vi "Configuration Tool Main.vi"() -> ()   [LabVIEW 2014, in "Advanced Configuration Tool.lvlib"]
doc: "This is the main VI for the configuration editor."
uses:
  Advanced Configuration Tool.lvlib
  Controls/StateCluster.ctl
  <vilib>/NI/Configuration Framework/Repository/NISE_CEF_Repository.lvclass
  <vilib>/NI/Configuration Framework/Node/NodeRef.ctl
  <vilib>/NI/Configuration Framework/Node/NISE_CEF_Node.lvclass
  <vilib>/NI/Configuration Framework/Node/UserEventRef.ctl
  <vilib>/NI/Configuration Framework/Controls/EventCluster.ctl
  Controls/AddMessage.ctl
  Controls/MoveMessage.ctl
  <vilib>/Utility/error.llb/DialogType.ctl
  <vilib>/NI/Configuration Framework/hierarchy repo/NISE_CEF_HierarchyRepo.lvclass
  Classes/My System/My System.lvclass
  <vilib>/NI/AMC/Read Termination Message.vi
  <vilib>/NI/AMC/Create Single Message.vi
  <vilib>/NI/AMC/Update Message Routing Info.vi
  <vilib>/NI/AMC/Globals.vi
  <vilib>/NI/AMC/Send Message.vi
  <vilib>/NI/AMC/AMC.lvlib
  <vilib>/NI/Configuration Framework/NISE_CEF_TreeControl.lvlib
  <vilib>/NI/Configuration Framework/serializable configuration/NISE_CEF_serializable configuration.lvclass
panel:
  in  "View":string(tree)
  in  "Exit":bool
  # "Configurator"
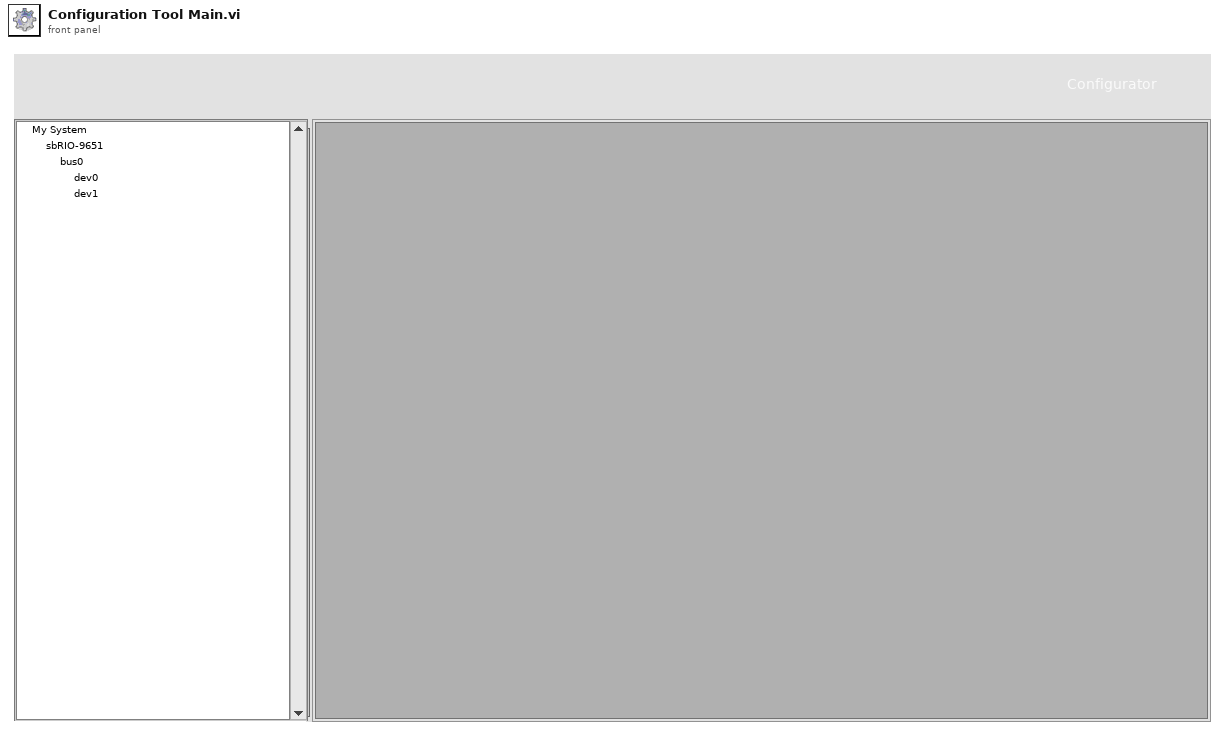
[diagram p1: front panel]
types:
  T1 = typedef "Advanced Configuration Tool.lvlib/StateCluster.ctl" = cluster{"repository":refnum<class "NISE_CEF_Repository.lvclass">, "root":T2, "unsaved changes":bool, "current path":path, "user event ref":T3, "glyph path":path, "classes path":path}
  T2 = typedef "NISE_CEF_Node.lvclass/NodeRef.ctl" = refnum<data-value>
  T3 = typedef "NISE_CEF_Node.lvclass/UserEventRef.ctl" = refnum<user-event>
  T4 = typedef "AMC.lvlib/Message Queue.ctl" = refnum<queue>
  T5 = typedef "Advanced Configuration Tool.lvlib/AddMessage.ctl" = cluster{"node type":string, "to add to":string}
  T6 = typedef "Advanced Configuration Tool.lvlib/MoveMessage.ctl" = cluster{"node ref":T2, "new parent":T2}
  T7 = enum32{"Invalid", "Standard", "Closed", "Hidden", "Minimized", "Maximized"}
  T8 = typedef "NISE_CEF_TreeControl.lvlib/EventCluster.ctl" = cluster{"command":string, "data":string}
  T9 = typedef "Advanced Configuration Tool.lvlib/FilePaths.ctl" = cluster{"glyphs":path, "classes":path}
  T10 = typedef "DialogType.ctl" = u16
  T11 = typedef "NISE_CEF_Node.lvclass/Summary.ctl" = cluster{"ID":string, "parent ID":string, "node type":string, "text":string, "additional text":string, "glyph":string, "depth":i32}
  T12 = typedef "LVPoint32TypeDef.ctl" = cluster{"Horizontal":i32, "Vertical":i32}
  T13 = cluster{"data name":string, "drag data":variant}[]
  T14 = typedef "NISE_CEF_Node.lvclass/NodeMenuOptions.ctl" = cluster{"removable":bool, "movable":bool, "duplicate":bool}
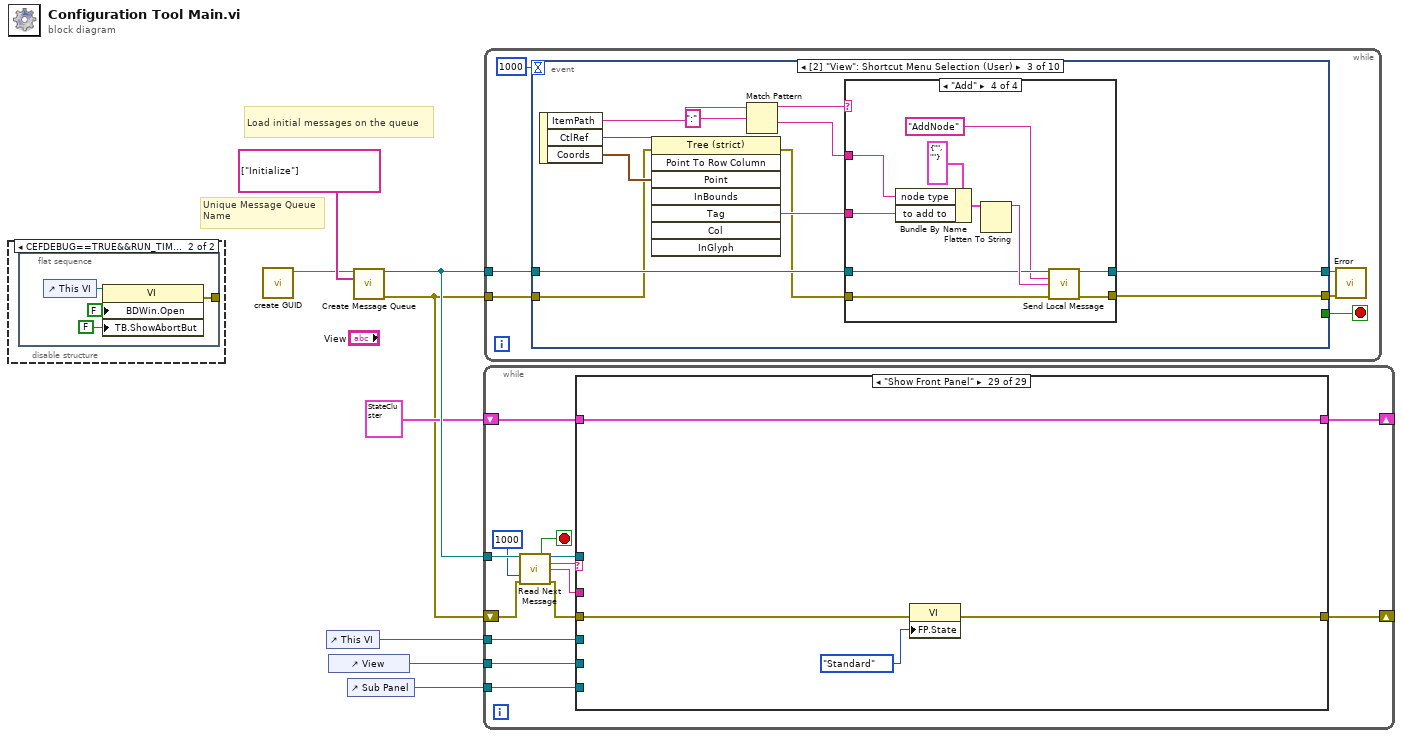
[diagram p0: block diagram]
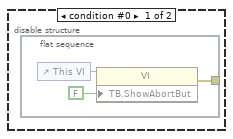
[diagram p2: hidden frame]
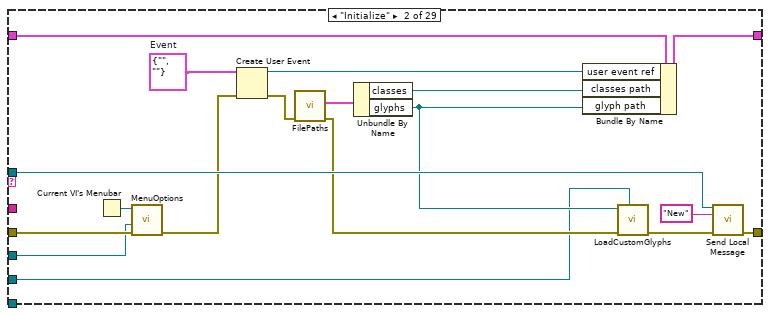
[diagram p4: hidden frame]
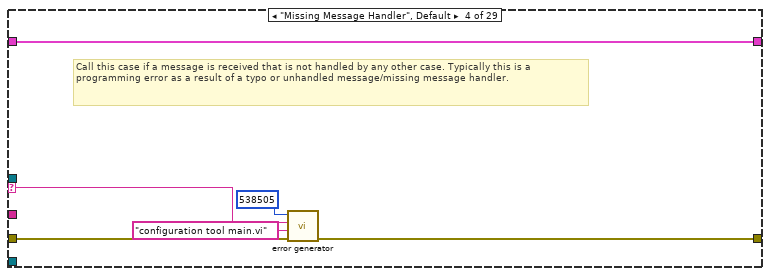
[diagram p6: hidden frame]
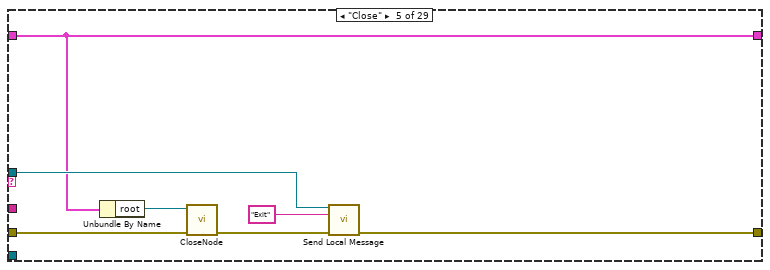
[diagram p7: hidden frame]
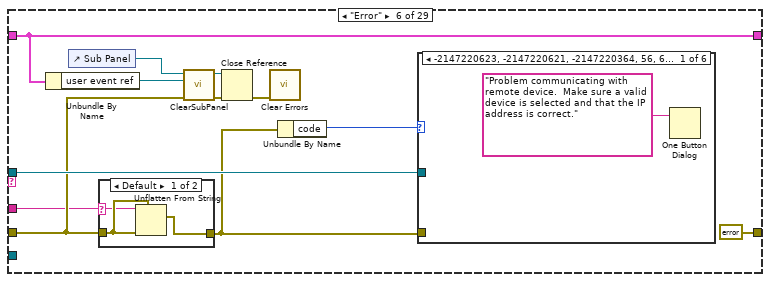
[diagram p8: hidden frame]
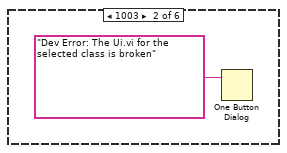
[diagram p10: hidden frame]
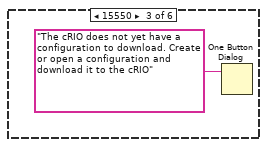
[diagram p11: hidden frame]
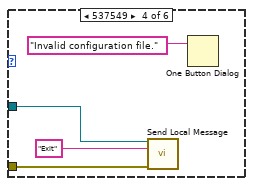
[diagram p12: hidden frame]
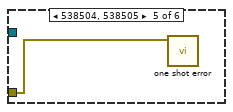
[diagram p13: hidden frame]
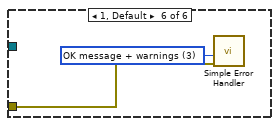
[diagram p14: hidden frame]
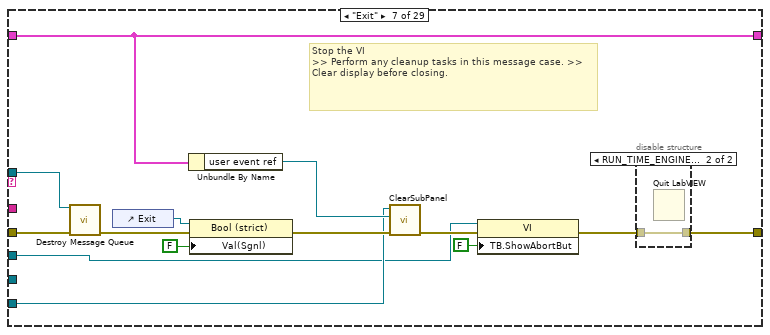
[diagram p15: hidden frame]
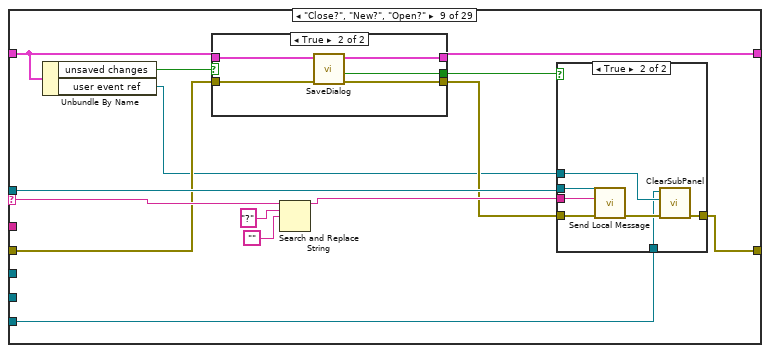
[diagram p18: hidden frame]
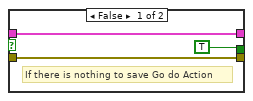
[diagram p19: hidden frame]
diagram:
  # "Unique Message Queue Name"
  # "Load initial messages on the queue"
  n1 = disable-structure shown="CEFDEBUG==TRUE&&RUN_TIME_ENGINE==False" {
    frame condition #0 {
      n2 = flat-sequence {
        tunnel: [w9] -> _
        frame #0 {
          n3 = control-ref of="This VI"() -> (w10:refnum<vi>)
          n4 = property class="VI"(reference=w10, "TB.ShowAbortBut"=FALSE ("Tool Bar:Show Abort Button")) -> (error out=w9:errorcluster)  [unwired: 1 in, 1 out]
        }
      }
    }
    frame condition #1 (active) {
      n5 = flat-sequence {
        tunnel: [w14] -> _
        frame #0 {
          n6 = control-ref of="This VI"() -> (w15:refnum<vi>)
          n7 = property class="VI"(reference=w15, "BDWin.Open"=FALSE ("Block Diagram Window:Open"), "TB.ShowAbortBut"=FALSE ("Tool Bar:Show Abort Button")) -> (error out=w14:errorcluster)  [unwired: 1 in, 1 out]
        }
      }
    }
  }
  n8 = call <vilib>:"create GUID.vi"() -> ("uuid"=w2:string)  [unwired: 11 in]
  n9 = control-ref of="This VI"() -> (w4:refnum<vi>)
  n10 = control-ref of="View"() -> (w3:refnum<vi>)
  n11 = control-ref of="Sub Panel"() -> (w1:refnum<vi>)
  n12 = call <vilib>:"Create Message Queue.vi"("message queue name"=w2, "initial message names"=string[] ["Initialize"]) -> ("message queue out"=w7:T4, "error out"=w5:errorcluster)  [unwired: 12 in]
  n13 = while "Message Processor" {
    shift-right: [w25] -> _
    shift-left: w5 -> [w24]
    tunnel: w7 -> [w23]
    shift-right: [w21] -> _
    shift-left: T1 {"repository"=refnum, "root"=refnum, "unsaved changes"=FALSE, "current path"=path "", "user event ref"=refnum, "glyph path"=path "", "classes path"=path ""} -> [w20]
    tunnel: w4 -> [w18]
    tunnel: w3 -> [w17]
    tunnel: w1 -> [w16]
    stop <- w29 stop-if-true
    n14 = call <vilib>:"Read Next Message.vi"("message queue in"=w23, "timeout (1 ms)"=1000, "error in"=w24) -> ("exit process?"=w29:bool, "message queue out"=w19:T4, "message name"=w28:string, "message value"=w27:string, "error out"=w26:errorcluster)  [unwired: 5 in, 3 out]
    n15 = case shown="\"Show Front Panel\"" w28 {
      selector: w28 -> [_ _ _ w54 _ _ _ _ w118 _ _ _ _ _ _ _ _ _ _ w366 _ _ _ _ _ _ _ _ _]
      tunnel: w27 -> [_ _ _ _ _ w65 _ _ _ _ _ _ _ w240 w272 _ w300 w332 w346 w364 w404 w428 _ _ w471 w493 _ _ _]
      tunnel: w26 -> [w31 w49 w51 w56 w59 w68 w104 w108 w111 w155 w166 w206 w232 w247 w273 w290 w301 w322 w345 w369 w406 w427 w452 w461 w470 w491 w496 w498 w503]
      tunnel: [w31 w45 w51 w55 w63 errorcluster {"status"=FALSE, "code"=0, "source"=""} ("error out") w97 w108 w122 w146 w162 w210 w234 w244 w260 w290 w304 w324 w349 w372 w410 w424 w447 w456 w467 w486 w496 w497 w502] -> w25
      tunnel: [w30 w40 w50 w57 w61 w73 w96 w107 w113 w159 w167 w213 w233 w241 w269 w289 w307 w315 w342 w373 w408 w421 w454 w460 w465 w482 w495 w500 w504] -> w21
      tunnel: w20 -> [w30 w41 w50 w57 w61 w73 w96 w107 w114 w158 w168 w208 w231 w242 w270 w289 w303 w320 w350 w373 w409 w429 w454 w460 w465 w494 w495 w500 w504]
      tunnel: w19 -> [_ w44 _ _ w62 w76 w103 _ w121 w160 w164 w209 _ w243 w265 _ w291 _ _ w367 _ _ _ _ w466 w485 _ _ _]
      tunnel: w18 -> [_ w32 _ _ _ _ w92 _ _ _ _ _ _ _ _ _ _ _ _ _ _ _ w439 _ _ _ _ _ _]
      tunnel: w17 -> [_ w33 _ _ _ _ _ _ _ _ _ _ _ _ _ _ _ w316 w343 w361 w401 w422 w440 _ _ _ _ _ _]
      tunnel: w16 -> [_ _ _ _ _ _ w94 _ w109 _ _ _ _ _ _ _ _ _ _ _ _ _ w437 w455 w462 _ _ _ _]
      frame "------------Generic Operations------------" {
        # "Dummy case to add a seperation in the Case Structure menu"
      }
      frame "Initialize" {
        w35 = T8 {"command"="", "data"=""}  # Event
        n16 = Current VI's Menubar() -> (w48:refnum<k9>)
        n17 = call "MenuOptions.vi"("error in"=w49, "VI ref"=w32, "menu ref in"=w48) -> ("error out"=w39:errorcluster)  [unwired: 7 in, 1 out]
        n18 = Create User Event(user event datatype=w35, error in=w39) -> (user event=w34:refnum<user-event>, error out=w38:errorcluster)
        n19 = call "FilePaths.vi"("error in"=w38) -> ("error out"=w43:errorcluster, "paths"=w42:T9)  [unwired: 9 in]
        n20 = Unbundle By Name(w42) -> ("classes"=w37:path, "glyphs"=w36:path)
        n21 = Bundle By Name(cluster=w41, "user event ref"=w34, "classes path"=w37, "glyph path"=w36) -> (w40:T1)
        n22 = call <vilib>:"LoadCustomGlyphs.vi"("tree ref"=w33, "error in"=w43, "glyph directory"=w36) -> ("error out"=w46:errorcluster)  [unwired: 8 in]
        n23 = call <vilib>:"Send Local Message.vi"("message queue in"=w44, "message name"="New" ("Message Name"), "error in"=w46) -> ("error out"=w45:errorcluster)  [unwired: 10 in, 2 out]
      }
      frame "", "Idle" {
      }
      frame "Missing Message Handler", Default {
        # "Call this case if a message is received that is not handled by any other case. Typically this is a programming error as a result of a typo or unhandled message/missing message handler."
        n24 = call <vilib>:"error generator.vi"("error in"=w56, "source"="configuration tool main.vi", "append error message"=w54, "error code (0)"=538505) -> ("error out"=w55:errorcluster)  [unwired: 5 in]
      }
      frame "Close" {
        n25 = Unbundle By Name(w61) -> ("root"=w60:T2)
        n26 = call <vilib>:"CloseNode.vi"("error in"=w59, "node ref"=w60) -> ("error out"=w58:errorcluster)  [unwired: 9 in]
        n27 = call <vilib>:"Send Local Message.vi"("message queue in"=w62, "message name"="Exit", "error in"=w58) -> ("error out"=w63:errorcluster)  [unwired: 10 in, 2 out]
      }
      frame "Error" {
        n28 = Unbundle By Name(w73) -> ("user event ref"=w71:T3)
        n29 = control-ref of="Sub Panel"() -> (w72:refnum<vi>)
        n30 = case shown="Default" w65 {
          selector: w65 -> [w78 _]
          tunnel: w68 -> [w79 w80]
          tunnel: [w77 w80] -> w67
          frame Default {
            n31 = Unflatten From String(type=w79, binary string=w78, error in (no error)=w79) -> (value=w77:errorcluster)  [unwired: 2 in, 2 out]
          }
          frame "" {
          }
        }
        n32 = call <vilib>:"ClearSubPanel.vi"("error in"=w68, "user event ref"=w71, "sub panel ref in"=w72) -> ("error out"=w70:errorcluster, "sub panel ref out"=w69:refnum<vi>)  [unwired: 7 in]
        n33 = Close Reference(reference=w69, error in (no error)=w70) -> (error out=w66:errorcluster)
        n34 = call <vilib>:"Clear Errors.vi"("error in (no error)"=w66) -> ()  [unwired: 5 in, 2 out]
        n35 = Unbundle By Name(w67) -> ("code"=w74:i32)
        n36 = case shown="-2147220623, -2147220621, -2147220364, 56, 63" w74 {
          tunnel: w76 -> [_ _ _ w86 _ _]
          tunnel: w67 -> [_ _ _ w85 w88 w90]
          frame -2147220623, -2147220621, -2147220364, 56, 63 {
            n37 = One Button Dialog(message="Problem communicating with remote device.  Make sure a valid device is selected and that the IP address is correct.") -> ()  [unwired: 1 in, 1 out]
          }
          frame 1003 {
            n38 = One Button Dialog(message="Dev Error: The Ui.vi for the selected class is broken") -> ()  [unwired: 1 in, 1 out]
          }
          frame 15550 {
            n39 = One Button Dialog(message="The cRIO does not yet have a configuration to download. Create or open a configuration and download it to the cRIO") -> ()  [unwired: 1 in, 1 out]
          }
          frame 537549 {
            n40 = call <vilib>:"Send Local Message.vi"("message queue in"=w86, "message name"="Exit", "error in"=w85) -> ()  [unwired: 10 in, 3 out]
            n41 = One Button Dialog(message="Invalid configuration file.") -> ()  [unwired: 1 in, 1 out]
          }
          frame 538504, 538505 {
            n42 = call <vilib>:"one shot error.vi"("error in"=w88) -> ()  [unwired: 11 in]
          }
          frame 1, Default {
            w89 = T10 3 items=["no dialog", "OK message", "continue or stop message", "OK message + warnings", "continue/stop + warnings"] ("type of dialog (OK msg:1)")
            n43 = call <vilib>:"Simple Error Handler.vi"("type of dialog (OK msg:1)"=w89, "error in (no error)"=w90) -> ()  [unwired: 8 out]
          }
        }
      }
      frame "Exit" {
        # "Stop the VI                                                                             >> Perform any cleanup tasks in this message case. >> Clear display before closing."
        n44 = call <vilib>:"Destroy Message Queue.vi"("message queue in"=w103, "error in"=w104) -> ("error out"=w100:errorcluster)  [unwired: 11 in, 2 out]
        n45 = control-ref of="Exit"() -> (w102:refnum<vi>)
        n46 = Unbundle By Name(w96) -> ("user event ref"=w95:T3)
        n47 = property class="Bool (strict)"(reference=w102, error in=w100, "Val(Sgnl)"=FALSE ("Exit")) -> (error out=w99:errorcluster)  [unwired: 1 out]
        n48 = call <vilib>:"ClearSubPanel.vi"("error in"=w99, "user event ref"=w95, "sub panel ref in"=w94) -> ("error out"=w98:errorcluster)  [unwired: 7 in, 1 out]
        n49 = property class="VI"(reference=w92, error in=w98, "TB.ShowAbortBut"=FALSE ("Tool Bar:Show Abort Button")) -> (error out=w93:errorcluster)  [unwired: 1 out]
        n50 = disable-structure shown="RUN_TIME_ENGINE==True" {
          disable-tunnel: [w105 w106] -> w97
          disable-tunnel: w93 -> [w105 w106]
          frame condition #0 (active) {
          }
          frame condition #1 {
            n51 = Quit LabVIEW() -> ()  [unwired: 1 in]
          }
        }
      }
      frame "------------Menu Operations--------------" {
        # "Dummy case to add a seperation in the Case Structure menu"
      }
      frame "Close?", "New?", "Open?" {
        n52 = Unbundle By Name(w114) -> ("unsaved changes"=w116:bool, "user event ref"=w110:T3)
        n53 = case shown="True" w116 {
          tunnel: [TRUE ("SaveFlag") w130] -> w115
          tunnel: w114 -> [w124 w129]
          tunnel: [w124 w128] -> w113
          tunnel: w111 -> [w123 w127]
          tunnel: [w123 w126] -> w112
          frame False {
            # "If there is nothing to save Go do Action"
          }
          frame True {
            n54 = call "SaveDialog.vi"("error in"=w127, "state in"=w129) -> ("error out"=w126:errorcluster, "new"=w130:bool, "state out"=w128:T1)  [unwired: 7 in]
          }
        }
        n55 = Search and Replace String(input string=w118, search string="?", replace string="") -> (result string=w117:string)  [unwired: 5 in, 3 out]
        n56 = case shown="True" w115 {
          tunnel: w112 -> [w131 w138]
          tunnel: [w131 w134] -> w122
          tunnel: w121 -> [_ w137]
          tunnel: w117 -> [_ w136]
          tunnel: w110 -> [_ w133]
          tunnel: w109 -> [_ w132]
          frame False {
          }
          frame True {
            n57 = call <vilib>:"Send Local Message.vi"("message queue in"=w137, "message name"=w136, "error in"=w138) -> ("error out"=w135:errorcluster)  [unwired: 10 in, 2 out]
            n58 = call <vilib>:"ClearSubPanel.vi"("error in"=w135, "user event ref"=w133, "sub panel ref in"=w132) -> ("error out"=w134:errorcluster)  [unwired: 7 in, 1 out]
          }
        }
      }
      frame "New" {
        n59 = Unbundle By Name(w158) -> ("classes path"=w157:path)
        n60 = call-dynamic "Initialize.vi"("error in"=w155, "path"=w157, "repository in"=refnum<class "NISE_CEF_HierarchyRepo.lvclass"> refnum ("NISE_CEF_HierarchyRepo.lvclass")) -> ("error out"=w156:errorcluster, "repository out"=w149:refnum<class "NISE_CEF_HierarchyRepo.lvclass">)  [unwired: 7 in]
        n61 = call-dynamic "Initialize.vi"("error in"=w156, "node in"=refnum<class "My System.lvclass"> refnum ("My System.lvclass")) -> ("error out"=w143:errorcluster, "data value reference"=w144:T2)  [unwired: 7 in, 1 out]
        n62 = call <vilib>:"NodetoID.vi"("error in"=w143, "node ref"=w144) -> ("error out"=w142:errorcluster, "ID"=w140:string)  [unwired: 8 in]
        n63 = call <vilib>:"Send Local Message.vi"("message queue in"=w160, "message name"="PopulateTree", "error in"=w142) -> ("message queue out"=w145:T4, "error out"=w151:errorcluster)  [unwired: 10 in, 1 out]
        n64 = Current VI's Menubar() -> (w150:refnum<k9>)
        n65 = call <vilib>:"NewMenu.vi"("error in"=w151, "menu ref in"=w150, "NISE_CEF_Repository in"=w149) -> ("error out"=w147:errorcluster, "NISE_CEF_Repository out"=w148:refnum<class "NISE_CEF_HierarchyRepo.lvclass">)  [unwired: 6 in, 1 out]
        n66 = Bundle By Name(cluster=w158, "current path"=path "", "unsaved changes"=FALSE, "repository"=w148, "root"=w144) -> (w159:T1)
        n67 = call <vilib>:"Send Local Message.vi"("message queue in"=w145, "message name"="ActivateNode", "message value"=w140, "error in"=w147) -> ("error out"=w146:errorcluster)  [unwired: 9 in, 2 out]
      }
      frame "Open" {
        n68 = in-place {
          in-place-border: w166 -> [w174]
          in-place-border: [w173] -> w163
          n69 = in-place-cluster #1(w168) -> ("current path"=w170:path, "repository"=w182:refnum<class "NISE_CEF_Repository.lvclass">, "root"=w178:T2)  [unwired: 1 out]
          n70 = call "generate default path.vi"("current file path"=w170) -> ("browse path"=w169:path)  [unwired: 10 in]
          n71 = call "FileDialog.vi"("error in"=w174, "start path"=w169) -> ("error out"=w175:errorcluster, "cancelled"=w176:bool, "selected path"=w172:path)  [unwired: 7 in]
          n72 = Compound Arithmetic op=OR(invert w176) -> (w177:bool)
          n73 = case shown="True" w177 {
            tunnel: w182 -> [w183 w195]
            tunnel: [w183 w193] -> w180
            tunnel: [w184 w191] -> w173
            tunnel: [w185 w190] -> w179
            tunnel: w172 -> [_ w188]
            tunnel: w175 -> [w184 w187]
            tunnel: w178 -> [w185 w186]
            frame False {
            }
            frame True {
              n74 = call-dynamic "Open.vi"("error in"=w187, "file path"=w188, "repository in"=w195) -> ("error out"=w192:errorcluster, "invalid?"=w189:bool, "repository out"=w194:refnum<class "NISE_CEF_Repository.lvclass">)  [unwired: 6 in]
              n75 = case shown="False" w189 {
                tunnel: w194 -> [w200 w203]
                tunnel: [w199 w203] -> w193
                tunnel: w192 -> [w198 w202]
                tunnel: [w197 w202] -> w191
                tunnel: [w196 w201] -> w190
                tunnel: w186 -> [_ w201]
                frame False {
                  n76 = call-dynamic "WriteTree.vi"("error in"=w198, "repository in"=w200) -> ("error out"=w197:errorcluster, "root"=w196:T2, "repository out"=w199:refnum<class "NISE_CEF_Repository.lvclass">)  [unwired: 7 in]
                }
                frame True {
                }
              }
            }
          }
          n77 = Select(t=w170, s=w173, f=w172) -> (s? t:f=w171:path)
          n78 = in-place-cluster #1("current path"=w171, "unsaved changes"=FALSE ("SaveFlag"), "repository"=w180, "root"=w179) -> (w167:T1)
        }
        n79 = call <vilib>:"Send Local Message.vi"("message queue in"=w164, "message name"="PopulateTree", "error in"=w163) -> ("error out"=w162:errorcluster)  [unwired: 10 in, 2 out]
      }
      frame "Save" {
        n80 = in-place {
          in-place-border: w206 -> [w218]
          in-place-border: [w217] -> w205
          in-place-border: [w215] -> w204
          n81 = in-place-cluster #2(w208) -> ("current path"=w216:path, "root"=w219:T2, "repository"=w220:refnum<class "NISE_CEF_Repository.lvclass">)
          n82 = Empty String/Path?(string/path=w216) -> (empty?=w215:bool)
          n83 = call-dynamic "ReadTree.vi"("error in"=w218, "root"=w219, "repository in"=w220) -> ("error out"=w217:errorcluster, "repository out"=w214:refnum<class "NISE_CEF_Repository.lvclass">)  [unwired: 7 in]
          n84 = in-place-cluster #2("current path"=w216, "root"=w219, "repository"=w214) -> (w207:T1)
        }
        n85 = case shown="True" w204 {
          tunnel: w207 -> [w224 w226]
          tunnel: [w223 w225] -> w213
          tunnel: [w222 w227] -> w211
          tunnel: w205 -> [w221 w228]
          frame False {
            n86 = call "Save.vi"("error in"=w221, "state in"=w224) -> ("error out"=w222:errorcluster, "state out"=w223:T1)  [unwired: 8 in]
          }
          frame True {
            # "Empty path use Dialog"
            n87 = call "SaveAs.vi"("error in"=w228, "state in"=w226) -> ("error out"=w227:errorcluster, "state out"=w225:T1)  [unwired: 7 in, 1 out]
          }
        }
        n88 = call <vilib>:"Send Local Message.vi"("message queue in"=w209, "message name"="PopulateTree", "error in"=w211) -> ("error out"=w210:errorcluster)  [unwired: 10 in, 2 out]
      }
      frame "SaveAs" {
        n89 = in-place {
          in-place-border: w232 -> [w236]
          in-place-border: [w235] -> w230
          n90 = in-place-cluster #3(w231) -> ("root"=w237:T2, "repository"=w239:refnum<class "NISE_CEF_Repository.lvclass">)
          n91 = call-dynamic "ReadTree.vi"("error in"=w236, "root"=w237, "repository in"=w239) -> ("error out"=w235:errorcluster, "repository out"=w238:refnum<class "NISE_CEF_Repository.lvclass">)  [unwired: 7 in]
          n92 = in-place-cluster #3("root"=w237, "repository"=w238) -> (w229:T1)
        }
        n93 = call "SaveAs.vi"("error in"=w230, "state in"=w229) -> ("error out"=w234:errorcluster, "state out"=w233:T1)  [unwired: 7 in, 1 out]
      }
      frame "Custom View" {
        n94 = in-place {
          in-place-border: w247 -> [w258]
          in-place-border: [w257] -> w245
          in-place-border: w240 -> [w248]
          n95 = in-place-cluster #4(w242) -> ("repository"=w252:refnum<class "NISE_CEF_Repository.lvclass">, "root"=w251:T2)
          n96 = call-dynamic "ReadTree.vi"("error in"=w258, "root"=w251, "repository in"=w252) -> ("error out"=w255:errorcluster, "repository out"=w254:refnum<class "NISE_CEF_Repository.lvclass">)  [unwired: 7 in]
          n97 = call-dynamic "CustomView.vi"("error in"=w255, "view name"=w248, "repository in"=w254) -> ("error out"=w256:errorcluster, "repository out"=w253:refnum<class "NISE_CEF_Repository.lvclass">)  [unwired: 7 in]
          n98 = call-dynamic "WriteTree.vi"("error in"=w256, "repository in"=w253) -> ("error out"=w257:errorcluster, "root"=w249:T2, "repository out"=w250:refnum<class "NISE_CEF_Repository.lvclass">)  [unwired: 7 in]
          n99 = in-place-cluster #4("repository"=w250, "root"=w249) -> (w241:T1)
        }
        n100 = call <vilib>:"Send Local Message.vi"("message queue in"=w243, "message name"="PopulateTree", "error in"=w245) -> ("error out"=w244:errorcluster)  [unwired: 10 in, 2 out]
      }
      frame "CustomFileMenu" {
        n101 = Unflatten From String(type=cluster{"ItemTag":string, string} {"ItemTag"="", ""} ("output cluster"), binary string=w272, error in (no error)=w273) -> (value=w259:cluster{"ItemTag":string, string}, error out=w268:errorcluster)  [unwired: 2 in, 1 out]
        n102 = Unbundle By Name(w270) -> ("repository"=w267:refnum<class "NISE_CEF_Repository.lvclass">)
        n103 = Unbundle(w259) -> ("ItemTag"=w264:string, w263:string)
        n104 = call-dynamic "HandleMenu.vi"("message queue"=w265, "error in"=w268, "Item Path"=w263, "ItemTag"=w264, "NISE_CEF_Repository in"=w267) -> ("error out"=w262:errorcluster, "handled?"=w261:bool, "NISE_CEF_Repository out"=w266:refnum<class "NISE_CEF_Repository.lvclass">)  [unwired: 4 in]
        n105 = case shown="False" w261 {
          tunnel: w262 -> [w277 w288]
          tunnel: [w278 w288] -> w260
          tunnel: w259 -> [w276 _]
          frame False {
            n106 = Unbundle(w276) -> ("ItemTag"=w275:string, w274:string)
            n107 = disable-structure shown="Default" {
              disable-tunnel: w277 -> [w284 w287]
              disable-tunnel: [w283 w287] -> w278
              disable-tunnel: w274 -> [w282 _]
              disable-tunnel: w275 -> [w281 _]
              frame condition #0 (active) {
                n108 = Concatenate Strings(w281, "::" ("string"), w282) -> (w280:string)
                n109 = call <vilib>:"error generator.vi"("error in"=w284, "source"="configuration tool main.vi", "append error message"=w280, "error code (0)"=538506) -> ("error out"=w283:errorcluster)  [unwired: 5 in]
              }
              frame condition #1 {
              }
            }
          }
          frame True {
          }
        }
        n110 = Bundle By Name(cluster=w270, "repository"=w266) -> (w269:T1)
      }
      frame "-------TreeControl Operations-----------" {
        # "Dummy case to add a seperation in the Case Structure menu"
      }
      frame "Select Target" {
        n111 = in-place {
          in-place-border: w301 -> [w311]
          in-place-border: w300 -> [w310]
          in-place-border: [w309] -> w297
          in-place-border: [w308] -> w298
          n112 = in-place-cluster #5(w303) -> ("repository"=w313:refnum<class "NISE_CEF_Repository.lvclass">)
          n113 = call-dynamic "GetClassPath.vi"("error in"=w311, "class name"=w310, "Repository in"=w313) -> ("error out"=w309:errorcluster, "class path"=w308:path, "Repository out"=w312:refnum<class "NISE_CEF_Repository.lvclass">)  [unwired: 6 in]
          n114 = in-place-cluster #5("repository"=w312) -> (w302:T1)
        }
        n115 = call <vilib>:"Get LV Class Default Value.vi"("error in (no error)"=w297, "class path"=w298) -> ("error out"=w296:errorcluster, "object"=w299:refnum<class>)  [unwired: 8 in]
        n116 = To More Specific Class(target class=refnum<class "NISE_CEF_Node.lvclass"> refnum ("Node.lvclass"), reference=w299, error in=w296) -> (specific class reference=w294:refnum<class "NISE_CEF_Node.lvclass">, error out=w293:errorcluster)
        n117 = call-dynamic "Initialize.vi"("error in"=w293, "node in"=w294) -> ("error out"=w292:errorcluster, "data value reference"=w306:T2)  [unwired: 7 in, 1 out]
        n118 = Bundle By Name(cluster=w302, "root"=w306) -> (w307:T1)
        n119 = call <vilib>:"Send Local Message.vi"("message queue in"=w291, "message name"="PopulateTree", "error in"=w292) -> ("error out"=w304:errorcluster)  [unwired: 10 in, 2 out]
      }
      frame "AddNode" {
        n120 = Unflatten From String(type=T5 {"node type"="", "to add to"=""} ("input cluster"), binary string=w332) -> (value=w330:T5)  [unwired: 3 in, 2 out]
        n121 = Unbundle By Name(w330) -> ("to add to"=w327:string, "node type"=w318:string)
        n122 = in-place {
          in-place-border: w322 -> [w338]
          in-place-border: [w337] -> w321
          in-place-border: w318 -> [w336]
          in-place-border: [w335] -> w317
          n123 = in-place-cluster #6(w320) -> ("repository"=w340:refnum<class "NISE_CEF_Repository.lvclass">)
          n124 = call-dynamic "GetClassPath.vi"("error in"=w338, "class name"=w336, "Repository in"=w340) -> ("error out"=w337:errorcluster, "class path"=w335:path, "Repository out"=w339:refnum<class "NISE_CEF_Repository.lvclass">)  [unwired: 6 in]
          n125 = in-place-cluster #6("repository"=w339) -> (w319:T1)
        }
        n126 = call <vilib>:"Get LV Class Default Value.vi"("error in (no error)"=w321, "class path"=w317) -> ("error out"=w333:errorcluster, "object"=w334:refnum<class>)  [unwired: 8 in]
        n127 = To More Specific Class(target class=refnum<class "NISE_CEF_Node.lvclass"> refnum ("Node.lvclass"), reference=w334, error in=w333) -> (specific class reference=w329:refnum<class "NISE_CEF_Node.lvclass">, error out=w326:errorcluster)
        n128 = call <vilib>:"AddNode.vi"("error in"=w326, "node in"=w329, "parent node ID"=w327) -> ("error out"=w325:errorcluster, "summary"=w323:T11[])  [unwired: 7 in]
        n129 = Bundle By Name(cluster=w319, "unsaved changes"=TRUE) -> (w315:T1)
        n130 = call <vilib>:"PopulateTreeSumary.vi"("error in"=w325, "array"=w323, "tree ref in"=w316) -> ("error out"=w324:errorcluster)  [unwired: 8 in]
      }
      frame "Duplicate" {
        n131 = call <vilib>:"IDtoNode.vi"("error in"=w345, "ID"=w346) -> ("error out"=w347:errorcluster, "invalid Id"=w344:bool, "node ref"=w348:T2)  [unwired: 7 in]
        n132 = case shown="False" w344 {
          tunnel: [w359 w360] -> w349
          tunnel: w348 -> [w358 _]
          tunnel: w347 -> [w355 w360]
          tunnel: w343 -> [w351 _]
          frame False {
            n133 = call <vilib>:"DuplicateNode.vi"("same parent?"=TRUE ("s"), "error in"=w355, "node ref in"=w358) -> ("error out"=w356:errorcluster, "new node ref"=w357:T2)  [unwired: 7 in]
            n134 = call <vilib>:"Summary.vi"("error in"=w356, "node self ref"=w357) -> ("error out"=w353:errorcluster, "summary"=w352:T11[])  [unwired: 8 in]
            n135 = call <vilib>:"PopulateTreeSumary.vi"("error in"=w353, "array"=w352, "tree ref in"=w351) -> ("error out"=w359:errorcluster)  [unwired: 8 in]
          }
          frame True {
          }
        }
        n136 = Bundle By Name(cluster=w350, "unsaved changes"=TRUE) -> (w342:T1)
      }
      frame "CustomMenuAction" {
        n137 = Match Pattern(string=w364, regular expression=":") -> (before substring=w363:string, after substring=w362:string)  [unwired: 1 in, 2 out]
        n138 = call <vilib>:"IDtoNode.vi"("error in"=w369, "ID"=w362) -> ("error out"=w370:errorcluster, "invalid Id"=w368:bool, "node ref"=w371:T2)  [unwired: 7 in]
        n139 = case shown="False" w368 {
          tunnel: [w376 w400] -> w372
          tunnel: w371 -> [w381 _]
          tunnel: w370 -> [w379 w400]
          tunnel: w367 -> [w380 _]
          tunnel: w366 -> [_ _]
          tunnel: w363 -> [w377 _]
          tunnel: w361 -> [w374 _]
          frame False {
            n140 = in-place {
              in-place-border: w380 -> [w398]
              in-place-border: w379 -> [w396]
              in-place-border: [w395] -> w375
              in-place-border: [w394] -> w378
              in-place-border: w377 -> [w393]
              in-place-border: w374 -> [w392]
              n141 = in-place-dvr #7(w381) -> (w399:refnum<class "NISE_CEF_Node.lvclass">)  [unwired: 1 out]
              n142 = call-dynamic "MenuHandler.vi"("tree control"=w392, "main message queue"=w398, "error in"=w396, "menu string"=w393, "NISE_CEF_Node in"=w399) -> ("error out"=w395:errorcluster, "Unhandled"=w394:bool, "NISE_CEF_Node out"=w397:refnum<class "NISE_CEF_Node.lvclass">)  [unwired: 4 in]
              n143 = in-place-dvr #7(w397) -> ()  [unwired: 2 out]
            }
            n144 = case shown="False" w378 {
              tunnel: w377 -> [_ w383]
              tunnel: [w382 w384] -> w376
              tunnel: w375 -> [w382 w385]
              frame False {
              }
              frame True {
                n145 = disable-structure shown="CEFDEBUG==TRUE" {
                  disable-tunnel: w385 -> [w388 w391]
                  disable-tunnel: [w387 w391] -> w384
                  disable-tunnel: w383 -> [w386 _]
                  frame condition #0 (active) {
                    n146 = call <vilib>:"error generator.vi"("error in"=w388, "source"="configuration tool main.vi", "append error message"=w386, "error code (0)"=538506) -> ("error out"=w387:errorcluster)  [unwired: 5 in]
                  }
                  frame condition #1 {
                  }
                }
              }
            }
          }
          frame True {
          }
        }
      }
      frame "RefreshNode" {
        # "Refreshes the node in the Tree               Sets the save flag to true                       This case can be called from the UIs of the nodes"
        n147 = call <vilib>:"IDtoNode.vi"("error in"=w406, "ID"=w404) -> ("error out"=w405:errorcluster, "invalid Id"=w402:bool, "node ref"=w403:T2)  [unwired: 7 in]
        n148 = case shown="False" w402 {
          tunnel: [w417 w419] -> w410
          tunnel: w405 -> [w413 w419]
          tunnel: w403 -> [w412 _]
          tunnel: w401 -> [w411 _]
          frame False {
            n149 = call <vilib>:"Summary.vi"("error in"=w413, "node self ref"=w412) -> ("error out"=w415:errorcluster, "summary"=w414:T11[])  [unwired: 8 in]
            n150 = call <vilib>:"RefreshSubTree.vi"("error in"=w415, "node information"=w414, "tree ref in"=w411) -> ("error out"=w418:errorcluster, "tree ref out"=w416:refnum<vi>)  [unwired: 7 in]
            n151 = Close Reference(reference=w416, error in (no error)=w418) -> (error out=w417:errorcluster)
          }
          frame True {
          }
        }
        n152 = Bundle By Name(cluster=w409, "unsaved changes"=TRUE ("SaveFlag")) -> (w408:T1)
      }
      frame "RemoveNode" {
        n153 = call <vilib>:"IDtoNode.vi"("error in"=w427, "ID"=w428) -> ("error out"=w426:errorcluster, "invalid Id"=w423:bool, "node ref"=w425:T2)  [unwired: 7 in]
        n154 = case shown="False" w423 {
          tunnel: w426 -> [w435 w436]
          tunnel: w425 -> [w434 _]
          tunnel: [w431 w436] -> w424
          tunnel: w422 -> [w430 _]
          frame False {
            n155 = call <vilib>:"RemoveNode.vi"("error in"=w435, "node"=w434) -> ("error out"=w432:errorcluster, "node ID"=w433:string)  [unwired: 8 in]
            n156 = call <vilib>:"ClearTreeNode.vi"("error in"=w432, "tag"=w433, "tree reference"=w430) -> ("error out"=w431:errorcluster)  [unwired: 8 in]
          }
          frame True {
          }
        }
        n157 = Bundle By Name(cluster=w429, "unsaved changes"=TRUE) -> (w421:T1)
      }
      frame "PopulateTree" {
        n158 = Unbundle By Name(w454) -> ("current path"=w445:path, "user event ref"=w446:T3, "root"=w450:T2)
        n159 = call <vilib>:"Summary.vi"("error in"=w452, "depth"=0 ("Depth"), "node self ref"=w450) -> ("error out"=w451:errorcluster, "summary"=w453:T11[])  [unwired: 7 in]
        n160 = call <vilib>:"Check if File or Folder Exists.vi"("path"=w445) -> ("file or folder exists?"=w443:bool, "dup path"=w444:path)  [unwired: 8 in, 1 out]
        n161 = Strip Path(path=w444) -> (name=w442:string)  [unwired: 1 out]
        n162 = call <vilib>:"RefreshEntireTree.vi"("calling VI in"=w439, "error in"=w451, "array"=w453, "tree ref in"=w440) -> ("error out"=w448:errorcluster)  [unwired: 7 in]
        n163 = Select(t=w442, s=w443, f="Advanced Configurator Sample Project") -> (s? t:f=w438:string)
        n164 = property class="VI"(reference=w439, "Front Panel.Title"=w438) -> ()  [unwired: 1 in, 2 out]
        n165 = call <vilib>:"ClearSubPanel.vi"("error in"=w448, "user event ref"=w446, "sub panel ref in"=w437) -> ("error out"=w447:errorcluster)  [unwired: 7 in, 1 out]
      }
      frame "CleansubPanel" {
        n166 = Unbundle By Name(w460) -> ("user event ref"=w459:T3)
        n167 = call <vilib>:"ClearSubPanel.vi"("error in"=w461, "user event ref"=w459, "sub panel ref in"=w455) -> ("error out"=w458:errorcluster, "sub panel ref out"=w457:refnum<vi>)  [unwired: 7 in]
        n168 = Close Reference(reference=w457, error in (no error)=w458) -> (error out=w456:errorcluster)
      }
      frame "ActivateNode" {
        n169 = Unbundle By Name(w465) -> ("user event ref"=w464:T3)
        n170 = call <vilib>:"IDtoNode.vi"("error in"=w470, "ID"=w471) -> ("error out"=w463:errorcluster, "invalid Id"=w469:bool, "node ref"=w468:T2)  [unwired: 7 in]
        n171 = case shown="False" w469 {
          tunnel: w468 -> [w478 _]
          tunnel: [w479 w480] -> w467
          tunnel: w463 -> [w476 w480]
          tunnel: w466 -> [w474 _]
          tunnel: w464 -> [w475 _]
          tunnel: w462 -> [w472 _]
          frame False {
            n172 = call <vilib>:"ClearSubPanel.vi"("error in"=w476, "user event ref"=w475, "sub panel ref in"=w472) -> ("error out"=w477:errorcluster, "sub panel ref out"=w473:refnum<vi>)  [unwired: 7 in]
            n173 = call <vilib>:"LoadNodeUI.vi"("user event out"=w475, "error in"=w477, "sub panel ref in"=w473, "main queue"=w474, "node"=w478) -> ("error out"=w479:errorcluster)  [unwired: 6 in]
          }
          frame True {
          }
        }
      }
      frame "Move" {
        n174 = Unflatten From String(type=T6 {"node ref"=refnum, "new parent"=refnum} ("Cluster"), binary string=w493, error in (no error)=w491) -> (value=w490:T6, error out=w489:errorcluster)  [unwired: 2 in, 1 out]
        n175 = Unbundle By Name(w490) -> ("node ref"=w484:T2, "new parent"=w483:T2)
        n176 = call <vilib>:"MoveNode.vi"("error in"=w489, "new parent"=w483, "node"=w484) -> ("error out"=w487:errorcluster)  [unwired: 8 in]
        n177 = Bundle By Name(cluster=w494, "unsaved changes"=TRUE) -> (w482:T1)
        n178 = call <vilib>:"Send Local Message.vi"("message queue in"=w485, "message name"="PopulateTree", "error in"=w487) -> ("error out"=w486:errorcluster)  [unwired: 10 in, 2 out]
      }
      frame "-------Custom SPI Operations-----------" {
      }
      frame "Hide Front Panel" {
        n179 = property class="VI"(error in=w498, "FP.State"=T7."Hidden" ("Front Panel Window:State")) -> (error out=w497:errorcluster)  [unwired: 1 in, 1 out]
      }
      frame "Show Front Panel" {
        n180 = property class="VI"(error in=w503, "FP.State"=T7."Standard" ("State")) -> (error out=w502:errorcluster)  [unwired: 1 in, 1 out]
      }
    }
  }
  n181 = while "User Interface Event Handler" {
    tunnel: w7 -> [w509]
    tunnel: w5 -> [w505]
    stop <- w508 stop-if-true
    n182 = event shown="[2] \"View\": Shortcut Menu Selection (User)" {
      selector: _ -> [_ _ _ _ _ _ _ _ _ _]
      dyn-events: _ -> [_ _ _ _ _ _ _ _ _ _]
      timeout: 1000 -> [_ _ _ _ _ _ _ _ _ _]
      tunnel: w509 -> [w512 w521 w546 w598 w626 w633 w662 w666 w676 w682]
      tunnel: [_ _ _ _ TRUE _ _ _ _ _] -> w508
      tunnel: [w512 w521 w543 w596 w622 w633 w659 w666 w674 w681] -> w507
      tunnel: [w511 w517 w542 w595 w623 w629 w658 w663 w672 w679] -> w506
      tunnel: w505 -> [w511 w520 w541 w597 w624 w632 w657 w665 w673 w680]
      event Timeout {
        # "Timeout code can be added here for autosave or Lock Screen"
        n183 = event-data() -> ()  [unwired: 1 in, 1 out]
      }
      event "View": Shortcut Menu Activation? {
        n184 = event-data() -> ("CtlRef"=w527:refnum<vi>, "Coords"=w526:T12, "MenuRef"=w523:refnum<k9>)  [unwired: 1 in]
        n185 = invoke class="Tree (strict)" method="Point To Row Column"(reference=w527, error in=w520, "Point"=w526) -> (error out=w519:errorcluster, "Tag"=w525:string)  [unwired: 5 in, 6 out]
        n186 = call <vilib>:"IDtoNode.vi"("error in"=w519, "ID"=w525) -> ("error out"=w515:errorcluster, "invalid Id"=w522:bool, "node ref"=w524:T2)  [unwired: 7 in]
        n187 = case shown="False" w522 {
          selector: w522 -> [_ w538]
          tunnel: w524 -> [w532 _]
          tunnel: w523 -> [w531 _]
          tunnel: [w530 _] -> w518
          tunnel: [w529 _] -> w516
          tunnel: w515 -> [w528 w539]
          tunnel: [w528 w539] -> w514
          tunnel: [_ w538] -> w513
          frame False {
            n188 = in-place {
              in-place-border: w531 -> [w535]
              in-place-border: [w533] -> w530
              n189 = in-place-dvr #8(w532) -> (w537:refnum<class "NISE_CEF_Node.lvclass">, w534:errorcluster)
              n190 = call-dynamic "ShortcutMenu.vi"("error in"=w534, "menu ref in"=w535, "node in"=w537) -> ("error out"=w533:errorcluster, "node out"=w536:refnum<class "NISE_CEF_Node.lvclass">)  [unwired: 6 in, 1 out]
              n191 = in-place-dvr #8(w536) -> (w529:errorcluster)  [unwired: 1 out]
            }
          }
          frame True {
          }
        }
        n192 = Merge Errors(w516, w518, w514) -> (w517:errorcluster)
        n193 = event-data("Discard?"=w513) -> ()  [unwired: 1 in, 1 out]
      }
      event "View": Shortcut Menu Selection (User) {
        n194 = event-data() -> ("ItemPath"=w545:string, "CtlRef"=w549:refnum<vi>, "Coords"=w550:T12)  [unwired: 1 in]
        n195 = invoke class="Tree (strict)" method="Point To Row Column"(reference=w549, error in=w541, "Point"=w550) -> (error out=w540:errorcluster, "Tag"=w544:string)  [unwired: 5 in, 6 out]
        n196 = Match Pattern(string=w545, regular expression=":") -> (before substring=w548:string, after substring=w547:string)  [unwired: 1 in, 2 out]
        n197 = case shown="\"Add\"" w548 {
          selector: w548 -> [w553 _ _ _]
          tunnel: w547 -> [_ _ _ w577]
          tunnel: w546 -> [w559 w566 w572 w579]
          tunnel: w544 -> [w555 w564 w570 w578]
          tunnel: [w556 w563 w569 w575] -> w543
          tunnel: [w557 w562 w567 w573] -> w542
          tunnel: w540 -> [w558 w561 w568 w574]
          frame Default {
            n198 = Concatenate Strings(w553, ":" ("string"), w555) -> (w552:string)
            n199 = call <vilib>:"Send Local Message.vi"("message queue in"=w559, "message name"="CustomMenuAction" ("Message Name"), "message value"=w552, "error in"=w558) -> ("message queue out"=w556:T4, "error out"=w557:errorcluster)  [unwired: 9 in, 1 out]
          }
          frame "Remove" {
            n200 = call <vilib>:"Send Local Message.vi"("message queue in"=w566, "message name"="RemoveNode" ("Message Name"), "message value"=w564, "error in"=w561) -> ("message queue out"=w563:T4, "error out"=w562:errorcluster)  [unwired: 9 in, 1 out]
          }
          frame "Duplicate" {
            n201 = call <vilib>:"Send Local Message.vi"("message queue in"=w572, "message name"="Duplicate" ("Message Name"), "message value"=w570, "error in"=w568) -> ("message queue out"=w569:T4, "error out"=w567:errorcluster)  [unwired: 9 in, 1 out]
          }
          frame "Add" {
            n202 = Bundle By Name(cluster=T5 {"node type"="", "to add to"=""} ("input cluster"), "node type"=w577, "to add to"=w578) -> (w580:T5)
            n203 = Flatten To String(anything=w580) -> (data string=w581:string)  [unwired: 3 in, 2 out]
            n204 = call <vilib>:"Send Local Message.vi"("message queue in"=w579, "message name"="AddNode" ("Message Name"), "message value"=w581, "error in"=w574) -> ("message queue out"=w575:T4, "error out"=w573:errorcluster)  [unwired: 9 in, 1 out]
          }
        }
      }
      event "View": Drop {
        n205 = event-data() -> ("CtlRef"=w601:refnum<vi>, "Coords"=w600:T12)  [unwired: 1 in]
        n206 = invoke class="Tree (strict)" method="Point To Row Column"(reference=w601, error in=w597, "Point"=w600) -> (reference out=w599:refnum<vi>, error out=w594:errorcluster, "Tag"=w591:string)  [unwired: 5 in, 5 out]
        n207 = call <vilib>:"ValidDragDrop.vi"("error in"=w594, "drag over"=w591, "tree ref in"=w599) -> ("error out"=w586:errorcluster, "accepted"=w589:bool, "drag"=w593:string, "tree ref out"=w603:refnum<vi>)  [unwired: 5 in]
        n208 = call <vilib>:"IDtoNode.vi"("error in"=w586, "ID"=w591) -> ("error out"=w587:errorcluster, "invalid Id"=w584:bool, "node ref"=w590:T2)  [unwired: 7 in]
        n209 = call <vilib>:"IDtoNode.vi"("error in"=w587, "ID"=w593) -> ("error out"=w585:errorcluster, "invalid Id"=w583:bool, "node ref"=w592:T2)  [unwired: 7 in]
        n210 = Compound Arithmetic op=AND(w589, invert w584, invert w583) -> (w588:bool)
        n211 = case shown="True" w588 {
          tunnel: w593 -> [_ w619]
          tunnel: w603 -> [_ w621]
          tunnel: [_ TRUE] -> w602
          tunnel: w591 -> [_ w617]
          tunnel: w598 -> [w605 w616]
          tunnel: [w605 w612] -> w596
          tunnel: [w604 w611] -> w595
          tunnel: w592 -> [_ w607]
          tunnel: w590 -> [_ w606]
          tunnel: w585 -> [w604 w608]
          frame False {
          }
          frame True {
            n212 = invoke class="Tree (strict)" method="Edit Tree Items.Move Item"(reference=w621, error in=w608, "tag"=w619, "New Parent"=w617) -> (error out=w609:errorcluster)  [unwired: 3 in, 6 out]
            n213 = Bundle By Name(cluster=T6 {"node ref"=refnum, "new parent"=refnum} ("Cluster"), "new parent"=w606, "node ref"=w607) -> (w615:T6)
            n214 = Flatten To String(anything=w615, error in (no error)=w609) -> (data string=w614:string, error out=w610:errorcluster)  [unwired: 2 in, 1 out]
            n215 = call <vilib>:"Send Local Message.vi"("message queue in"=w616, "message name"="Move", "message value"=w614, "error in"=w610) -> ("message queue out"=w612:T4, "error out"=w611:errorcluster)  [unwired: 9 in, 1 out]
          }
        }
        n216 = event-data("Accepted?"=w602) -> ()  [unwired: 1 in, 1 out]
      }
      event "Exit": Value Change {
        # "Exit the application                                           >> Stop this message generator loop    Cleaning errors if the other loop stop this one"
        n217 = event-data() -> ()  [unwired: 1 in, 1 out]
        n218 = call <vilib>:"Send Local Message.vi"("message queue in"=w626, "message name"="Close", "error in"=w624) -> ("message queue out"=w622:T4, "error out"=w627:errorcluster)  [unwired: 10 in, 1 out]
        n219 = call <vilib>:"Clear Errors.vi"("error in (no error)"=w627) -> ("error out"=w623:errorcluster)  [unwired: 5 in, 1 out]
      }
      event "View": Drag Starting? {
        n220 = event-data() -> ("Data"=w639:T13, "CtlRef"=w641:refnum<vi>, "Coords"=w640:T12)  [unwired: 1 in]
        n221 = invoke class="Tree (strict)" method="Point To Row Column"(reference=w641, error in=w632, "Point"=w640) -> (error out=w631:errorcluster, "Tag"=w638:string)  [unwired: 5 in, 6 out]
        n222 = call <vilib>:"IDtoNode.vi"("error in"=w631, "ID"=w638) -> ("error out"=w630:errorcluster, "invalid Id"=w637:bool, "node ref"=w636:T2)  [unwired: 7 in]
        n223 = case shown="False" w637 {
          tunnel: w636 -> [w649 _]
          tunnel: [w646 TRUE ("Removable")] -> w634
          tunnel: w630 -> [w645 w655]
          tunnel: [w642 w655] -> w629
          frame False {
            n224 = in-place {
              in-place-border: [w652] -> w648
              in-place-border: w645 -> [w651]
              in-place-border: [w650] -> w644
              n225 = in-place-dvr #9(w649) -> (w654:refnum<class "NISE_CEF_Node.lvclass">)  [unwired: 1 out]
              n226 = call-dynamic "EditOptions.vi"("error in"=w651, "node in"=w654) -> ("error out"=w650:errorcluster, "edit options"=w652:T14, "node out"=w653:refnum<class "NISE_CEF_Node.lvclass">)  [unwired: 6 in, 1 out]
              n227 = in-place-dvr #9(w653) -> (w643:errorcluster)  [unwired: 1 out]
            }
            n228 = Unbundle By Name(w648) -> ("movable"=w647:bool)
            n229 = Merge Errors(w643, w644) -> (w642:errorcluster)
            n230 = Not(x=w647) -> (.not. x?=w646:bool)
          }
          frame True {
          }
        }
        n231 = event-data("Data"=w639, "Drag Mode"=enum32{"copy or move", "copy only", "move only"}."move only", "Discard?"=w634) -> ()  [unwired: 1 in, 1 out]
      }
      event "View": Value Change {
        n232 = event-data() -> ("NewVal"=w660:string)  [unwired: 1 in]
        n233 = call <vilib>:"Send Local Message.vi"("message queue in"=w662, "message name"="ActivateNode" ("Message Name"), "message value"=w660, "error in"=w657) -> ("message queue out"=w659:T4, "error out"=w658:errorcluster)  [unwired: 9 in, 1 out]
      }
      event "View": event type 3.0.xa000003a {
        n234 = event-data() -> ("CtlRef"=w671:refnum<vi>, "Coords"=w668:T12)  [unwired: 1 in]
        n235 = invoke class="Tree (strict)" method="Point To Row Column"(reference=w671, error in=w665, "Point"=w668) -> (reference out=w670:refnum<vi>, error out=w664:errorcluster, "Tag"=w669:string)  [unwired: 5 in, 5 out]
        n236 = call <vilib>:"ValidDragDrop.vi"("error in"=w664, "drag over"=w669, "tree ref in"=w670) -> ("error out"=w663:errorcluster, "accepted"=w667:bool)  [unwired: 5 in, 2 out]
        n237 = event-data("Accepted?"=w667) -> ()  [unwired: 1 in, 1 out]
      }
      event Panel Close? {
        # "Intercepts the upper right close panel operation to allow a smooth shutdown as opposed to immediately killing the app."
        n238 = event-data() -> ()  [unwired: 1 in, 1 out]
        n239 = call <vilib>:"Send Local Message.vi"("message queue in"=w676, "message name"="Close?", "error in"=w673) -> ("message queue out"=w674:T4, "error out"=w672:errorcluster)  [unwired: 10 in, 1 out]
        n240 = event-data("Discard?"=TRUE) -> ()  [unwired: 1 in, 1 out]
      }
      event Menu Selection (User) {
        # "#USERCFG It is needed to add a Case for Every item on the menu"
        n241 = event-data() -> ("ItemTag"=w678:string, "ItemPath"=w683:string)  [unwired: 1 in]
        n242 = case shown="\"_File:_New\"" w683 {
          selector: w683 -> [_ _ _ _ _ w713]
          tunnel: w682 -> [w688 w693 w698 w703 w708 w721]
          tunnel: [w684 w689 w694 w699 w704 w718] -> w681
          tunnel: w680 -> [w686 w691 w696 w701 w706 w709]
          tunnel: [w685 w690 w695 w700 w705 w716] -> w679
          tunnel: w678 -> [_ _ _ _ _ w714]
          frame "_File:_New" {
            n243 = call <vilib>:"Send Local Message.vi"("message queue in"=w688, "message name"="New?" ("Message Name"), "error in"=w686) -> ("message queue out"=w684:T4, "error out"=w685:errorcluster)  [unwired: 10 in, 1 out]
          }
          frame "_File:_Open" {
            n244 = call <vilib>:"Send Local Message.vi"("message queue in"=w693, "message name"="Open?" ("Message Name"), "error in"=w691) -> ("message queue out"=w689:T4, "error out"=w690:errorcluster)  [unwired: 10 in, 1 out]
          }
          frame "_File:_Save" {
            n245 = call <vilib>:"Send Local Message.vi"("message queue in"=w698, "message name"="Save" ("Message Name"), "error in"=w696) -> ("message queue out"=w694:T4, "error out"=w695:errorcluster)  [unwired: 10 in, 1 out]
          }
          frame "_File:Save As..." {
            n246 = call <vilib>:"Send Local Message.vi"("message queue in"=w703, "message name"="SaveAs" ("Message Name"), "error in"=w701) -> ("message queue out"=w699:T4, "error out"=w700:errorcluster)  [unwired: 10 in, 1 out]
          }
          frame "_File:_Exit" {
            n247 = call <vilib>:"Send Local Message.vi"("message queue in"=w708, "message name"="Close?" ("Message Name"), "error in"=w706) -> ("message queue out"=w704:T4, "error out"=w705:errorcluster)  [unwired: 10 in, 1 out]
          }
          frame Default {
            n248 = Bundle("ItemTag"=w714, w713) -> (w712:cluster{"ItemTag":string, string})  [unwired: 1 in]
            n249 = Flatten To String(anything=w712, error in (no error)=w709) -> (data string=w711:string, error out=w710:errorcluster)  [unwired: 2 in, 1 out]
            n250 = call <vilib>:"Send Local Message.vi"("message queue in"=w721, "message name"="CleansubPanel", "error in"=w710) -> ("message queue out"=w720:T4, "error out"=w717:errorcluster)  [unwired: 10 in, 1 out]
            n251 = call <vilib>:"Send Local Message.vi"("message queue in"=w720, "message name"="CustomFileMenu" ("Message Name"), "message value"=w711, "error in"=w717) -> ("message queue out"=w718:T4, "error out"=w716:errorcluster)  [unwired: 9 in, 1 out]
          }
        }
      }
    }
    n252 = call "Error.vi"("error in (no error)"=w506, "message queue in"=w507) -> ()  [unwired: 9 in, 1 out]
  }
